vi "Left Auto V.3.0.vi"(11 "Desired Angle":dbl) -> (3 "Stop":bool)   [LabVIEW 2017]
uses:
  Robot Global Data V.3.0.vi
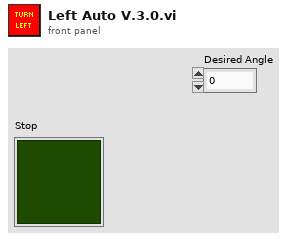
[diagram p1: front panel]
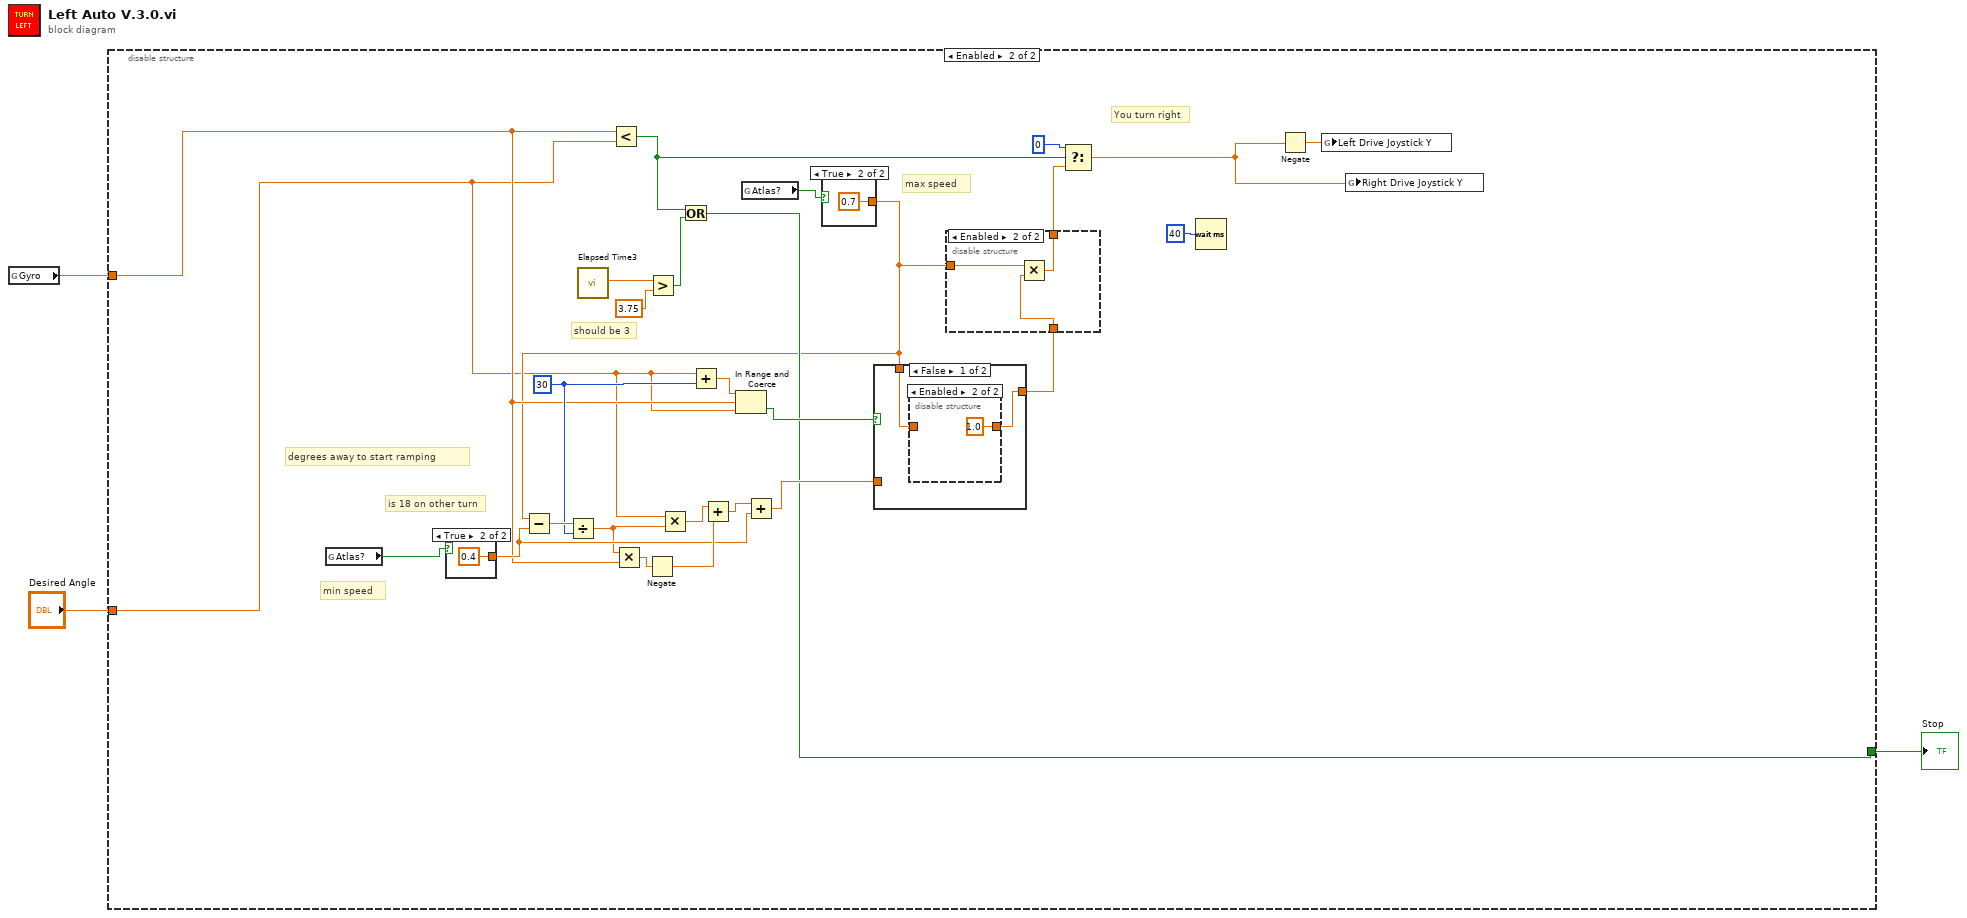
[diagram p0: block diagram]
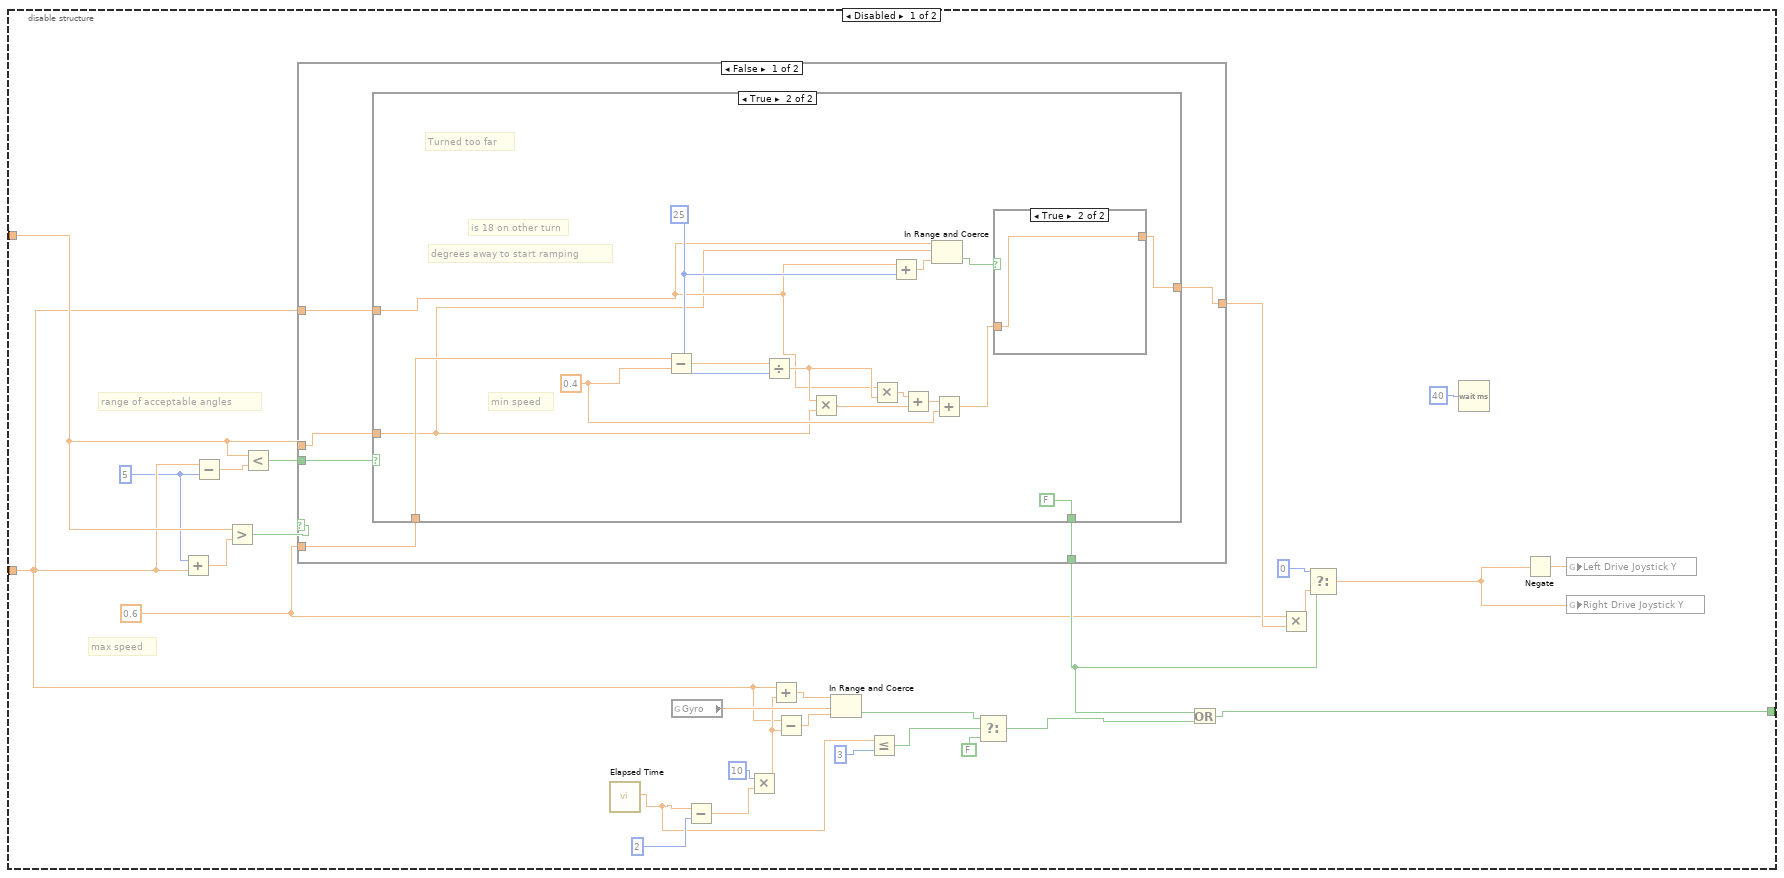
[diagram p2: hidden frame]
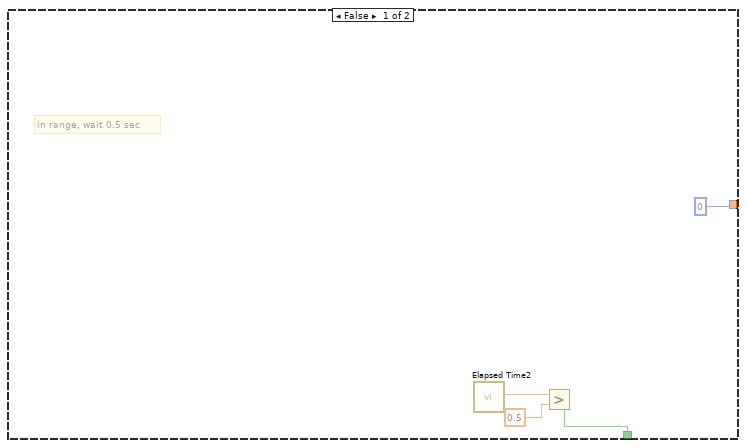
[diagram p3: hidden frame]
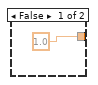
[diagram p4: hidden frame]
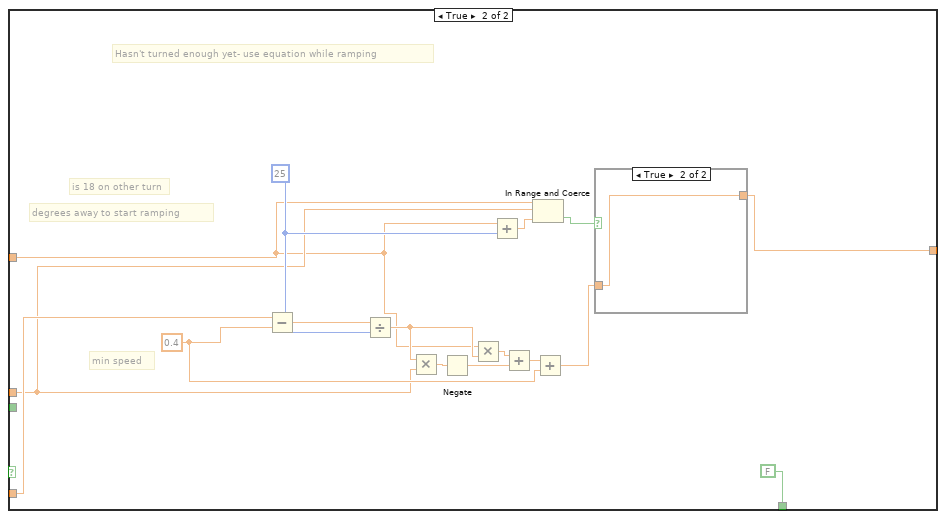
[diagram p5: hidden frame]
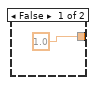
[diagram p6: hidden frame]
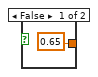
[diagram p8: hidden frame]
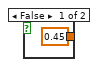
[diagram p9: hidden frame]
diagram:
  n1 = global read "Robot Global Data V.3.0.vi" "Gyro"() -> (w3:dbl)
  n2 = disable-structure shown="Enabled" {
    disable-tunnel: w3 -> [w21 w87]
    disable-tunnel: "Desired Angle" -> [w7 w78]
    disable-tunnel: [w4 w86] -> w1
    frame Disabled {
      w6 = 5
      w5 = 0.6
      # "range of acceptable angles"
      # "max speed"
      n3 = Add(x=w6, y=w7) -> (x+y=w27:dbl)
      n4 = Subtract(x=w7, y=w6) -> (x-y=w25:dbl)
      n5 = Greater?(x=w21, y=w27) -> (0:w26:bool)
      n6 = Less?(x=w21, y=w25) -> (x < y?=w24:bool)
      n7 = case shown="False" w26 {
        tunnel: w24 -> [w37 _]
        tunnel: [w38 FALSE] -> w23
        tunnel: w21 -> [w33 w61]
        tunnel: w5 -> [w34 w63]
        tunnel: w7 -> [w35 w60]
        tunnel: [w36 w62] -> w22
        frame False {
          n8 = case shown="True" w37 {
            tunnel: [w40 FALSE] -> w38
            tunnel: [0 w47] -> w36
            tunnel: w35 -> [_ w46]
            tunnel: w34 -> [_ w45]
            tunnel: w33 -> [_ w44]
            frame False {
              # "in range, wait 0.5 sec"
              n9 = call "Elapsed Time2"() -> ("Elapsed Time (s)"=w42:dbl)  [unwired: 12 in, 7 out]
              n10 = Greater?(x=w42, y=0.5) -> (0:w40:bool)
            }
            frame True {
              w49 = 25
              w48 = 0.4
              # "is 18 on other turn"
              # "degrees away to start ramping"
              # "min speed"
              # "Turned too far"
              n11 = Subtract(x=w45, y=w48) -> (x-y=w55:dbl)
              n12 = Divide(x=w55, y=w49) -> (x/y=w56:dbl)
              n13 = Multiply(x=w56, y=w44) -> (x*y=w43:dbl)
              n14 = Multiply(x=w46, y=w56) -> (x*y=w52:dbl)
              n15 = Add(x=w46, y=w49) -> (x+y=w50:dbl)
              n16 = Add(x=w52, y=w43) -> (x+y=w53:dbl)
              n17 = In Range and Coerce(upper limit=w46, x=w44, lower limit=w50) -> (In Range?=w51:bool)  [unwired: 1 out]
              n18 = Add(x=w53, y=w48) -> (x+y=w54:dbl)
              n19 = case shown="True" w51 {
                tunnel: w54 -> [_ w59]
                tunnel: [1.0 w59] -> w47
                frame False {
                }
                frame True {
                }
              }
            }
          }
        }
        frame True {
          w65 = 25
          w64 = 0.4
          # "is 18 on other turn"
          # "degrees away to start ramping"
          # "min speed"
          # "Hasn't turned enough yet- use equation while ramping"
          n20 = Subtract(x=w63, y=w64) -> (x-y=w73:dbl)
          n21 = Divide(x=w73, y=w65) -> (x/y=w74:dbl)
          n22 = Multiply(x=w74, y=w61) -> (x*y=w68:dbl)
          n23 = Negate(x=w68) -> (-x=w70:dbl)
          n24 = Multiply(x=w60, y=w74) -> (x*y=w69:dbl)
          n25 = Add(x=w60, y=w65) -> (x+y=w66:dbl)
          n26 = Add(x=w69, y=w70) -> (x+y=w71:dbl)
          n27 = In Range and Coerce(upper limit=w60, x=w61, lower limit=w66) -> (In Range?=w67:bool)  [unwired: 1 out]
          n28 = Add(x=w71, y=w64) -> (x+y=w72:dbl)
          n29 = case shown="True" w67 {
            tunnel: w72 -> [_ w77]
            tunnel: [1.0 w77] -> w62
            frame False {
            }
            frame True {
            }
          }
        }
      }
      n30 = call "Elapsed Time"() -> ("Elapsed Time (s)"=w13:dbl)  [unwired: 12 in, 7 out]
      n31 = global read "Robot Global Data V.3.0.vi" "Gyro"() -> (w18:dbl)
      n32 = Subtract(x=w13, y=2) -> (x-y=w15:dbl)
      n33 = Multiply(x=10, y=w15) -> (x*y=w14:dbl)
      n34 = Add(x=w7, y=w14) -> (x+y=w20:dbl)
      n35 = Subtract(x=w7, y=w14) -> (x-y=w19:dbl)
      n36 = In Range and Coerce(upper limit=w20, x=w18, lower limit=w19) -> (In Range?=w10:bool)  [unwired: 1 out]
      n37 = Less Or Equal?(x=w13, y=3) -> (x <= y?=w11:bool)
      n38 = Select(t=w10, s=w11, f=FALSE) -> (s? t:f=w8:bool)
      n39 = Or(x=w23, y=w8) -> (x .or. y?=w4:bool)
      n40 = Multiply(x=w5, y=w22) -> (x*y=w30:dbl)
      n41 = Select(t=0, s=w23, f=w30) -> (s? t:f=w28:dbl)
      n42 = Wait (ms)(milliseconds to wait=u32 40) -> ()  [unwired: 1 out]
      n43 = Negate(x=w28) -> (-x=w29:dbl)
      n44 = global write "Robot Global Data V.3.0.vi" "Left Drive Joystick Y"(w29) -> ()
      n45 = global write "Robot Global Data V.3.0.vi" "Right Drive Joystick Y"(w28) -> ()
    }
    frame Enabled {
      w94 = 30
      # "is 18 on other turn"
      # "should be 3"
      # "degrees away to start ramping"
      # "max speed"
      # "min speed"
      # "You turn right"
      n46 = global read "Robot Global Data V.3.0.vi" "Atlas?"() -> (w84:bool)
      n47 = case shown="True" w84 {
        tunnel: [0.45 0.4] -> w98
        frame False {
        }
        frame True {
        }
      }
      n48 = call "Elapsed Time3"() -> ("Elapsed Time (s)"=w91:dbl)  [unwired: 12 in, 7 out]
      n49 = Less?(x=w87, y=w78) -> (x < y?=w89:bool)
      n50 = Greater?(x=w91, y=3.75) -> (0:w90:bool)
      n51 = Or(x=w89, y=w90) -> (x .or. y?=w86:bool)
      n52 = Add(x=w78, y=w94) -> (x+y=w79:dbl)
      n53 = In Range and Coerce(upper limit=w79, x=w87, lower limit=w78) -> (In Range?=w102:bool)  [unwired: 1 out]
      n54 = global read "Robot Global Data V.3.0.vi" "Atlas?"() -> (w83:bool)
      n55 = case shown="True" w83 {
        tunnel: [0.65 0.7] -> w80
        frame False {
        }
        frame True {
        }
      }
      n56 = Subtract(x=w80, y=w98) -> (x-y=w95:dbl)
      n57 = Divide(x=w95, y=w94) -> (x/y=w93:dbl)
      n58 = Multiply(x=w93, y=w87) -> (x*y=w101:dbl)
      n59 = Negate(x=w101) -> (-x=w99:dbl)
      n60 = Multiply(x=w78, y=w93) -> (x*y=w100:dbl)
      n61 = Add(x=w100, y=w99) -> (x+y=w97:dbl)
      n62 = Add(x=w97, y=w98) -> (x+y=w96:dbl)
      n63 = case shown="False" w102 {
        tunnel: w96 -> [_ w117]
        tunnel: [w114 w117] -> w81
        tunnel: w80 -> [w113 _]
        frame False {
          n64 = disable-structure shown="Enabled" {
            disable-tunnel: [w115 1.0] -> w114
            disable-tunnel: w113 -> [w115 _]
            frame Disabled {
            }
            frame Enabled {
            }
          }
        }
        frame True {
        }
      }
      n65 = disable-structure shown="Enabled" {
        disable-tunnel: [w105 w108] -> w82
        disable-tunnel: w81 -> [w105 w107]
        disable-tunnel: w80 -> [_ w106]
        frame Disabled {
        }
        frame Enabled {
          n66 = Multiply(x=w106, y=w107) -> (x*y=w108:dbl)
        }
      }
      n67 = Select(t=0, s=w89, f=w82) -> (s? t:f=w85:dbl)
      n68 = Wait (ms)(milliseconds to wait=u32 40) -> ()  [unwired: 1 out]
      n69 = Negate(x=w85) -> (-x=w92:dbl)
      n70 = global write "Robot Global Data V.3.0.vi" "Left Drive Joystick Y"(w92) -> ()
      n71 = global write "Robot Global Data V.3.0.vi" "Right Drive Joystick Y"(w85) -> ()
    }
  }
  "Stop" <- w1
